vi "Create J1939 Addon.vi"(7 "Merge Path (.dat)":path, 8 "error in (no error)":errorcluster, 10 "Configuration":T4 {"J1939 XNET Settings"."Termination" items=["Off", "On"]; "J1939 Monitor Settings"."Name" format="%.0x"; "Devices"."J1939 Monitor Settings"."Name" format="%.0x"}, 11 "CustomDevices":refnum<k24>) -> (0 "error out":errorcluster, 3 "CustomDevices out":refnum<k24>)   [LabVIEW 2023, in "J1939 System Definition API.lvlib"]
uses:
  J1939 System Definition API.lvlib
  Addon/Addon Shared/Types/XNET Settings.ctl
  Addon/Addon Shared/Types/Monitor Settings.ctl
  Types/Add Item - Frame Cluster.ctl
  NationalInstruments.VeriStand.SystemDefinitionAPI
  Types/Remove Frame Action.ctl
  Addon/Addon Shared/SubVIs/Constants.vi
  <vilib>/NI/NI VeriStand Advanced SysDef API/_SubVIs/SysDef.Search.Target.vi
  <vilib>/NI/NI VeriStand Advanced SysDef API/_SubVIs/SysDef.Search.GUID.vi
  <vilib>/NI/NI VeriStand Advanced SysDef API/_SubVIs/SysDef.Search.Name.vi
  <vilib>/NI/NI VeriStand Advanced SysDef API/_SubVIs/SysDef.Property.Set.String.vi
  SubVIs/Add Frames.vi
  SubVIs/Add Device.vi
  SubVIs/Add DTC.vi
  J1939 System Definition API Support.lvlib
  Addon/Addon Shared/J1939 Addon Shared.lvlib
  <vilib>/NI/NI VeriStand Custom Device Import and Export Tool/ImportExport.lvlib
  <vilib>/NI/NI VeriStand Advanced SysDef API/SysDef API/Advanced System Definition.lvlib
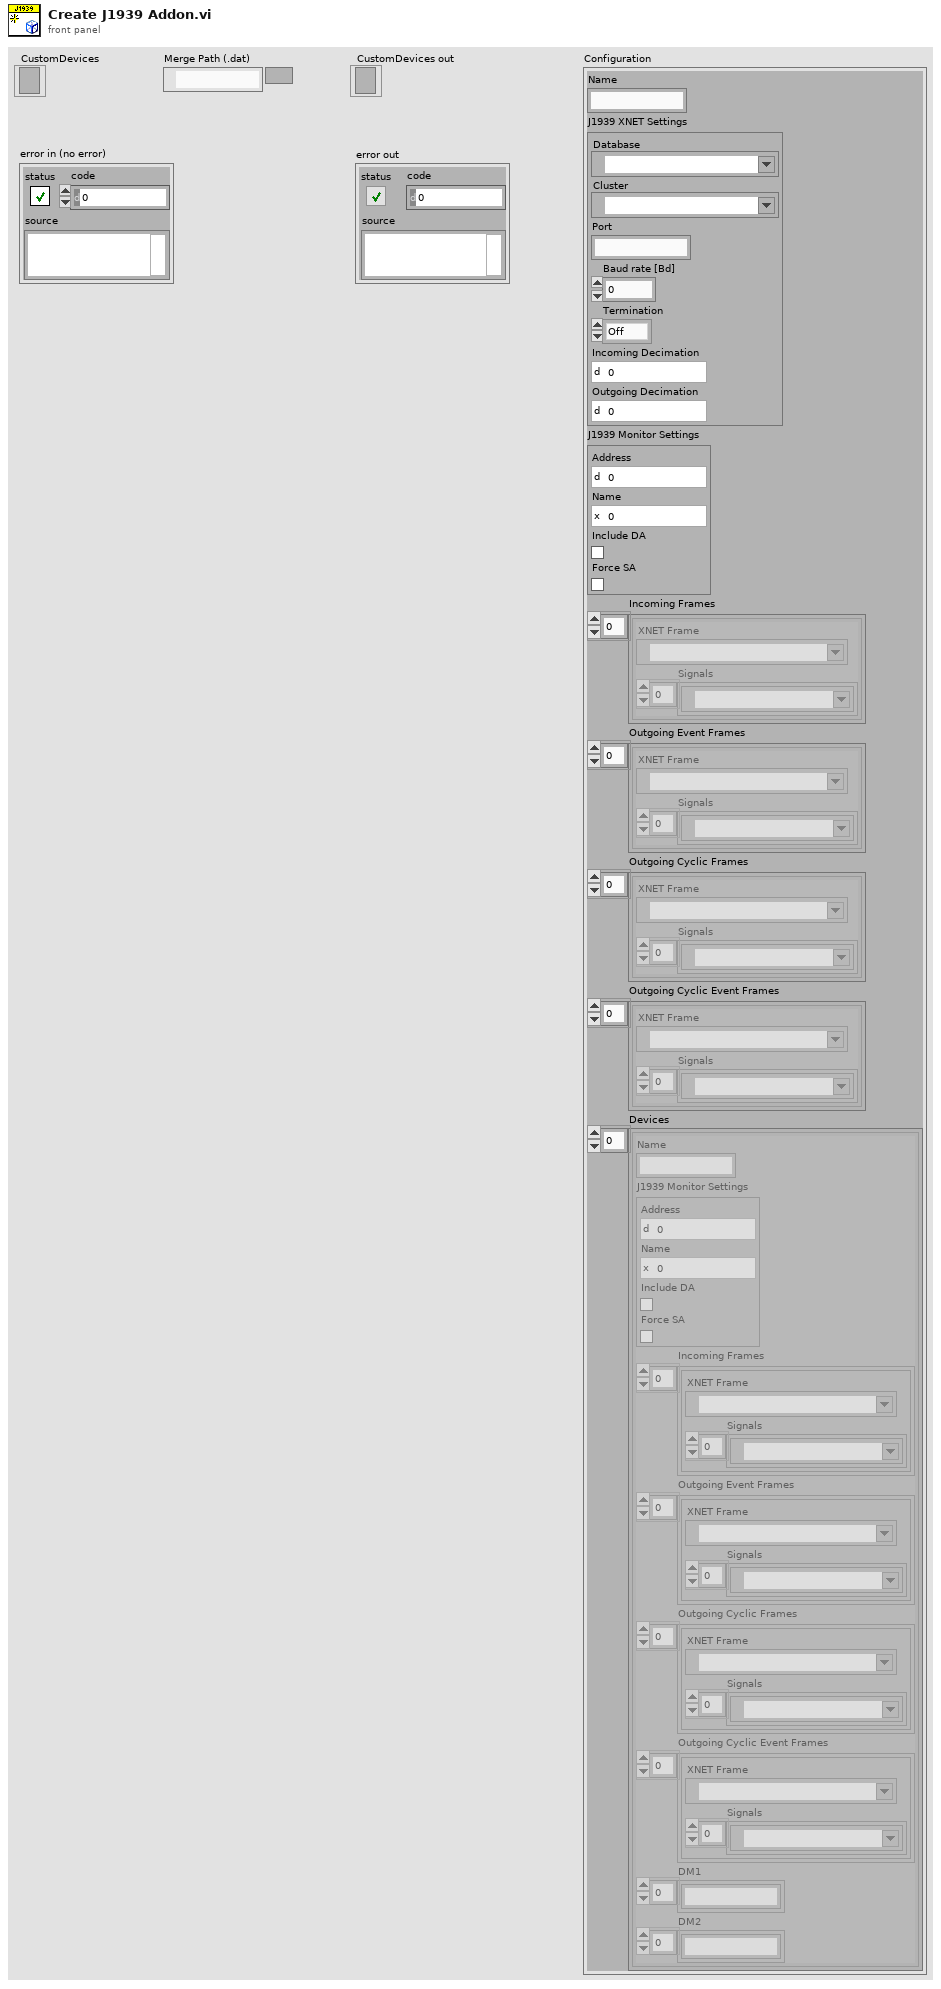
[diagram p1: front panel]
types:
  T1 = typedef "J1939 Addon Shared.lvlib/XNET Settings.ctl" = cluster{"Database":refnum<k21>, "Cluster":refnum<k21>, "Port":string, "Baud rate [Bd]":u32, "Termination":u32, "Incoming Decimation":u32, "Outgoing Decimation":u32}
  T2 = typedef "J1939 Addon Shared.lvlib/Monitor Settings.ctl" = cluster{"Address":u8, "Name":u64, "Include DA":bool, "Force SA":bool}
  T3 = typedef "J1939 System Definition API Support.lvlib/Add Item - Frame Cluster.ctl" = cluster{"XNET Frame":refnum<k21>, "Signals":refnum<k21>[]}
  T4 = cluster{"Name":string, "J1939 XNET Settings":T1, "J1939 Monitor Settings":T2, "Incoming Frames":T3[], "Outgoing Event Frames":T3[], "Outgoing Cyclic Frames":T3[], "Outgoing Cyclic Event Frames":T3[], "Devices":cluster{"Name":string, "J1939 Monitor Settings":T2, "Incoming Frames":T3[], "Outgoing Event Frames":T3[], "Outgoing Cyclic Frames":T3[], "Outgoing Cyclic Event Frames":T3[], "DM1":string[], "DM2":string[]}[]}
  T5 = typedef "J1939 System Definition API Support.lvlib/Remove Frame Action.ctl" = enum16{"Incoming", "Outgoing Event", "Outgoing Cyclic", "Outgoing Cyclic Event"}
  T6 = cluster{"Name":string, "J1939 Monitor Settings":T2, "Incoming Frames":T3[], "Outgoing Event Frames":T3[], "Outgoing Cyclic Frames":T3[], "Outgoing Cyclic Event Frames":T3[], "DM1":string[], "DM2":string[]}[]
  T7 = typedef "Custom Device API.lvlib/Custom Device Item Ref.ctl" = u64
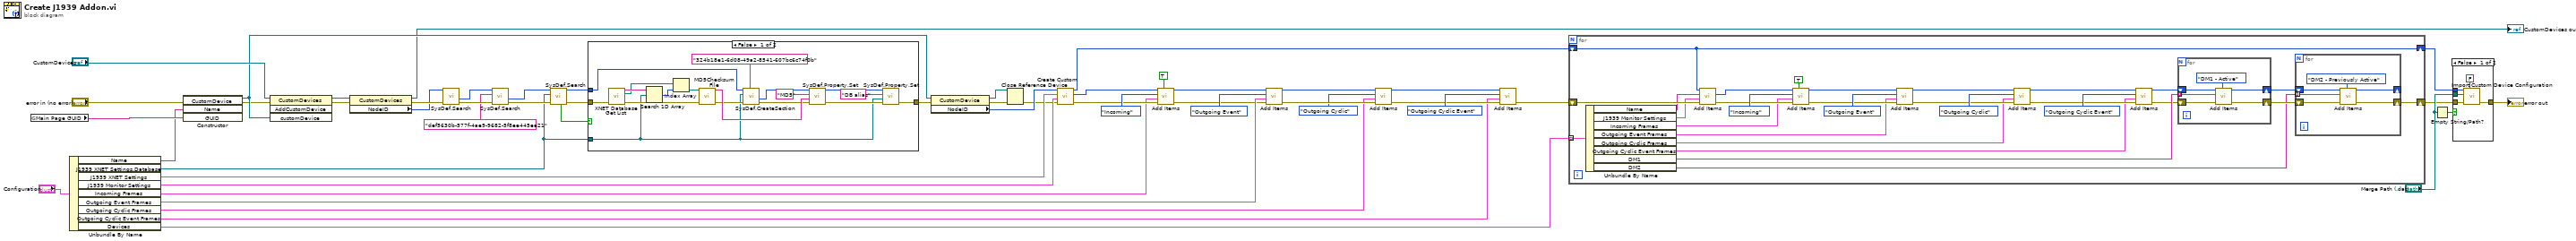
[diagram p0: block diagram]
diagram:
  n1 = global read "Constants.vi" "Main Page GUID"() -> (w40:string)
  n2 = Unbundle By Name("Configuration") -> ("Name"=w39:string, "J1939 XNET Settings.Database"=w14:refnum<k21>, "J1939 XNET Settings"=w46:T1, "J1939 Monitor Settings"=w45:T2, "Incoming Frames"=w44:T3[], "Outgoing Event Frames"=w43:T3[], "Outgoing Cyclic Frames"=w7:T3[], "Outgoing Cyclic Event Frames"=w2:T3[], "Devices"=w41:T6)
  n3 = constructor class="CustomDevice"(error in="error in (no error)", "Name"=w39, "GUID"=w40) -> (reference out=w37:refnum<k24>, error out=w36:errorcluster)  [unwired: 2 in, 3 out]
  n4 = invoke class="CustomDevices" method="AddCustomDevice"(reference="CustomDevices", error in=w36, "customDevice"=w37) -> (reference out=w28:refnum<k24>, error out=w25:errorcluster)  [unwired: 1 in, 2 out]
  n5 = property class="CustomDevices"(reference=w28, error in=w25) -> (reference out=→"CustomDevices out":refnum<k24>, error out=w24:errorcluster, "NodeID"=w23:u64)
  n6 = call-poly <vilib>:"SysDef.Search.vi"("error in (no error)"=w24, "nodeID"=w23) -> ("error out"=w22:errorcluster, "Value out"=w21:u64)  [unwired: 6 in, 2 out]
  n7 = call-poly <vilib>:"SysDef.Search.vi"("error in (no error)"=w22, "GUID"="def5630b-577f-4ae9-9682-5f8ee445ee21" ("string"), "nodeID"=w21) -> ("error out"=w19:errorcluster, "Value out"=w18:u64)  [unwired: 5 in, 2 out]
  n8 = call-poly <vilib>:"SysDef.Search.vi"("error in (no error)"=w19, "Name"=w14, "nodeID"=w18) -> ("error out"=w15:errorcluster, "nodeID out"=w16:u64, "Found?"=w17:bool)  [unwired: 5 in, 1 out]
  n9 = case shown="False" w17 {
    tunnel: [w62 w72] -> w26
    tunnel: w15 -> [w60 w72]
    tunnel: w16 -> [w61 _]
    tunnel: w14 -> [w54 _]
    frame False {
      n10 = call <vilib>:"XNET Database Get List.vi"("error in (no error)"=w60) -> ("array of alias"=w58:string[], "array of filepath"=w56:path[], "error out"=w59:errorcluster)  [unwired: 12 in]
      n11 = Search 1D Array(1D array=w58, element=w54) -> (index of element=w57:i32)  [unwired: 1 in]
      n12 = Index Array(array=w56, index=w57) -> (element=w55:path)
      n13 = call <vilib>:"MD5Checksum File.vi"("error in (no error)"=w59, "Path"=w55) -> ("error out"=w70:errorcluster, "MD5 message-digest"=w71:string)  [unwired: 8 in]
      n14 = call <vilib>:"SysDef.CreateSection.vi"("GUID"="324b18e1-6d08-49a2-8541-607bc6c74f0b" ("GUID (Default Section)"), "error in (no error)"=w70, "Name"=w54, "nodeID"=w61) -> ("error out"=w64:errorcluster, "New NodeID"=w63:u64)  [unwired: 4 in, 2 out]
      n15 = call-poly <vilib>:"SysDef.Property.Set.vi"("error in (no error)"=w64, "Value"=w71, "Property Name"="MD5", "nodeID"=w63) -> ("error out"=w65:errorcluster, "nodeID out"=w66:u64)  [unwired: 6 in]
      n16 = call-poly <vilib>:"SysDef.Property.Set.vi"("error in (no error)"=w65, "Value"=w54, "Property Name"="DB alias", "nodeID"=w66) -> ("error out"=w62:errorcluster)  [unwired: 6 in, 1 out]
    }
    frame True {
    }
  }
  n17 = property class="CustomDevice"(reference=w37, error in=w26) -> (reference out=w11:refnum<k24>, error out=w13:errorcluster, "NodeID"=w34:u64)
  n18 = Close Reference(reference=w11, error in (no error)=w13) -> (error out=w12:errorcluster)
  n19 = call "Create Custom Device.vi"("error in (no error)"=w12, "J1939 Monitor Settings"=w45, "J1939 XNET Settings"=w46, "Device Item Ref in"=w34) -> ("error out"=w48:errorcluster, "Monitor Ref out"=w53:T7, "Device Item Ref out"=w49:T7)  [unwired: 5 in]
  n20 = call-poly "Add Items.vi"("Add Info?"=TRUE, "error in (no error)"=w48, "Frames"=w44, "Action"=Remove_Frame_Action."Incoming", "Section Ref in"=w53) -> ("error out"=w42:errorcluster, "Section Ref out"=w51:T7)  [unwired: 5 in]
  n21 = call-poly "Add Items.vi"("error in (no error)"=w42, "Frames"=w43, "Action"=Remove_Frame_Action."Outgoing Event", "Section Ref in"=w51) -> ("error out"=w10:errorcluster, "Section Ref out"=w9:T7)  [unwired: 6 in]
  n22 = call-poly "Add Items.vi"("error in (no error)"=w10, "Frames"=w7, "Action"=Remove_Frame_Action."Outgoing Cyclic", "Section Ref in"=w9) -> ("error out"=w5:errorcluster, "Section Ref out"=w4:T7)  [unwired: 6 in]
  n23 = call-poly "Add Items.vi"("error in (no error)"=w5, "Frames"=w2, "Action"=Remove_Frame_Action."Outgoing Cyclic Event", "Section Ref in"=w4) -> ("error out"=w3:errorcluster)  [unwired: 6 in, 1 out]
  n24 = for {
    tunnel: w41 -> [w92] mode=indexing
    shift-right: [w85] -> w31
    shift-left: w3 -> [w101]
    shift-right: [w84] -> w29
    shift-left: w49 -> [w84]
    n25 = Unbundle By Name(w92) -> ("Name"=w91:string, "J1939 Monitor Settings"=w90:T2, "Incoming Frames"=w89:T3[], "Outgoing Event Frames"=w88:T3[], "Outgoing Cyclic Frames"=w80:T3[], "Outgoing Cyclic Event Frames"=w74:T3[], "DM1"=w87:string[], "DM2"=w86:string[])
    n26 = call-poly "Add Items.vi"("error in (no error)"=w101, "J1939 Monitor Settings"=w90, "Name"=w91, "NodeID"=w84) -> ("error out"=w96:errorcluster, "Device Ref out"=w97:T7)  [unwired: 6 in]
    n27 = call-poly "Add Items.vi"("Add Info?"=TRUE, "error in (no error)"=w96, "Frames"=w89, "Action"=Remove_Frame_Action."Incoming", "Section Ref in"=w97) -> ("error out"=w95:errorcluster, "Section Ref out"=w99:T7)  [unwired: 5 in]
    n28 = call-poly "Add Items.vi"("error in (no error)"=w95, "Frames"=w88, "Action"=Remove_Frame_Action."Outgoing Event", "Section Ref in"=w99) -> ("error out"=w82:errorcluster, "Section Ref out"=w81:T7)  [unwired: 6 in]
    n29 = call-poly "Add Items.vi"("error in (no error)"=w82, "Frames"=w80, "Action"=Remove_Frame_Action."Outgoing Cyclic", "Section Ref in"=w81) -> ("error out"=w77:errorcluster, "Section Ref out"=w78:T7)  [unwired: 6 in]
    n30 = call-poly "Add Items.vi"("error in (no error)"=w77, "Frames"=w74, "Action"=Remove_Frame_Action."Outgoing Cyclic Event", "Section Ref in"=w78) -> ("error out"=w76:errorcluster, "Section Ref out"=w75:T7)  [unwired: 6 in]
    n31 = for {
      shift-right: [w104] -> w94
      shift-left: w75 -> [w106]
      shift-right: [w103] -> w93
      shift-left: w76 -> [w105]
      tunnel: w87 -> [w102] mode=indexing
      n32 = call-poly "Add Items.vi"("DTC Type"=enum8{"DM1 - Active", "DM2 - Previously Active"}."DM1 - Active", "error in (no error)"=w105, "Name"=w102, "Device Ref in"=w106) -> ("error out"=w103:errorcluster, "Device Ref out"=w104:T7)  [unwired: 6 in]
    }
    n33 = for {
      shift-right: [w110] -> _
      shift-left: w94 -> [w112]
      shift-right: [w109] -> w85
      shift-left: w93 -> [w111]
      tunnel: w86 -> [w108] mode=indexing
      n34 = call-poly "Add Items.vi"("DTC Type"=enum8{"DM1 - Active", "DM2 - Previously Active"}."DM2 - Previously Active", "error in (no error)"=w111, "Name"=w108, "Device Ref in"=w112) -> ("error out"=w109:errorcluster, "Device Ref out"=w110:T7)  [unwired: 6 in]
    }
  }
  n35 = Empty String/Path?(string/path="Merge Path (.dat)") -> (empty?=w32:bool)
  n36 = case shown="False" w32 {
    tunnel: [w118 w119] -> w30
    tunnel: w31 -> [w117 w119]
    tunnel: w29 -> [w116 _]
    tunnel: "Merge Path (.dat)" -> [w115 _]
    frame False {
      n37 = call <vilib>:"Import Custom Device Configuration.vi"("Overwrite Existing?"=FALSE, "error in (no error)"=w117, "Path"=w115, "NodeID"=w116) -> ("error out"=w118:errorcluster)  [unwired: 5 in, 2 out]
    }
    frame True {
    }
  }
  "error out" <- w30
